vi "DynamicMotionMagicVoltage SetControl.vi"(0 "UseTimesync":bool, 1 "StopSendingOtherRequests":bool=TRUE, 2 "Position":dbl, 3 "Velocity":dbl, 4 "Acceleration":dbl, 5 "Jerk":dbl, 6 "EnableFOC":bool=TRUE, 7 "error in":errorcluster, 8 "FeedForward":dbl, 9 "Slot":i32, 10 "OverrideBrakeDurNeutral":bool, 11 "LimitForwardMotion":bool, 12 "LimitReverseMotion":bool, 13 "IgnoreHardwareLimits":bool, 18 "Update Frequency (Hz)":dbl=100.0) -> (20 "DeviceReference Out":T1, 27 "error out":errorcluster)   [LabVIEW 2023]
doc: "Requests Motion Magic® to target a final position using a motion profile. This dynamic request allows runtime changes to Cruise Velocity, Acceleration, and Jerk. Users can optionally provide a voltage feedforward. This control requires use of a CANivore.\nMotion Magic® produces a motion profile in real-time while attempting to honor the specified Cruise Velocity, Acceleration, and (optional) Jerk. This control mode does not use the Expo_kV or Expo_kA configs.\nTarget position can be changed on-the-fly and Motion Magic® will do its best to adjust the profile. This control mode is voltage-based, so relevant closed-loop gains will use Volts for the numerator."
uses:
  Users/test.DESKTOP-CORY/Documents/PhoenixProLabVIEWGeneration/CopyDown/DeviceReference.ctl
panel:
  in  "DeviceReference":T1
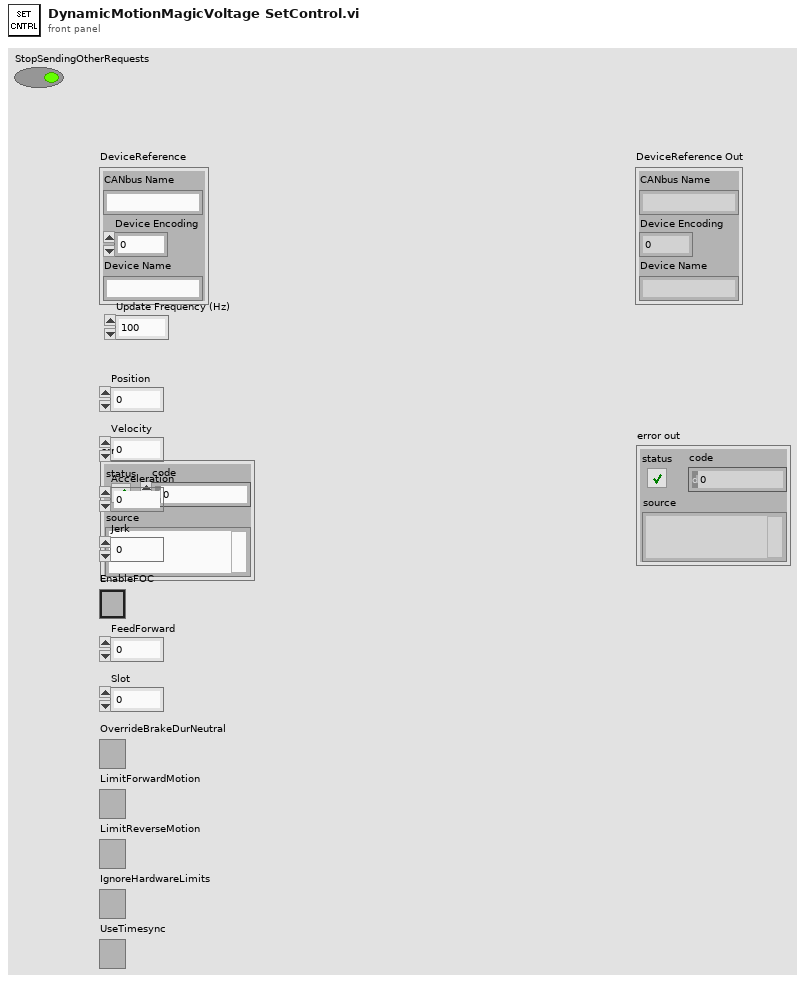
[diagram p1: front panel]
types:
  T1 = typedef "DeviceReference.ctl" = cluster{"CANbus Name":string, "Device Encoding":u32, "Device Name":string}
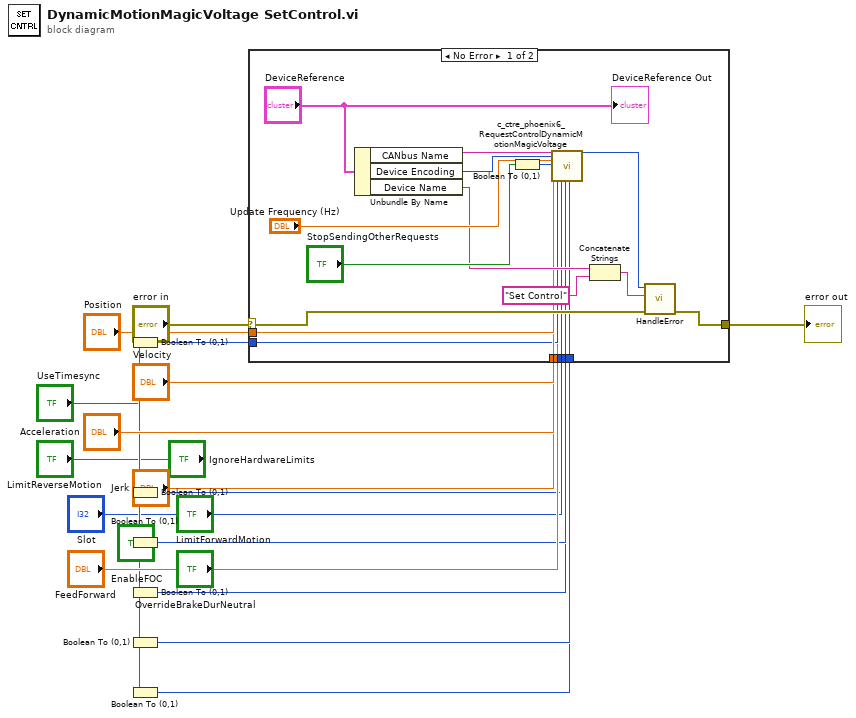
[diagram p0: block diagram]
diagram:
  n1 = Boolean To (0,1)(Boolean="EnableFOC") -> (0, 1=w13:i16)
  n2 = Boolean To (0,1)(Boolean="OverrideBrakeDurNeutral") -> (0, 1=w9:i16)
  n3 = Boolean To (0,1)(Boolean="LimitForwardMotion") -> (0, 1=w7:i16)
  n4 = Boolean To (0,1)(Boolean="LimitReverseMotion") -> (0, 1=w5:i16)
  n5 = Boolean To (0,1)(Boolean="IgnoreHardwareLimits") -> (0, 1=w3:i16)
  n6 = Boolean To (0,1)(Boolean="UseTimesync") -> (0, 1=w1:i16)
  n7 = case shown="No Error" "error in" {
    selector: "error in" -> [w37 w45]
    tunnel: [w36 w45] -> w19
    tunnel: "Position" -> [w32 _]
    tunnel: "Velocity" -> [w31 _]
    tunnel: "Acceleration" -> [w30 _]
    tunnel: "Jerk" -> [w29 _]
    tunnel: w13 -> [w28 _]
    tunnel: "FeedForward" -> [w27 _]
    tunnel: "Slot" -> [w26 _]
    tunnel: w9 -> [w25 _]
    tunnel: w7 -> [w24 _]
    tunnel: w5 -> [w23 _]
    tunnel: w3 -> [w22 _]
    tunnel: w1 -> [w21 _]
    frame No Error {
      n8 = Unbundle By Name("DeviceReference") -> ("CANbus Name"=w43:string, "Device Encoding"=w42:u32, "Device Name"=w35:string)
      n9 = Boolean To (0,1)(Boolean="StopSendingOtherRequests") -> (0, 1=w39:i16)
      n10 = call <vilib>:"c_ctre_phoenix6_RequestControlDynamicMotionMagicVoltage.vi"("String 2"=w43, "Numeric 2"=w42, "Numeric 3"="Update Frequency (Hz)", "Numeric 4"=w39, "Numeric 5"=w32, "Numeric 6"=w31, "Numeric 7"=w30, "Numeric 8"=w29, "Numeric 9"=w28, "Numeric 10"=w27, "Numeric 11"=w26, "Numeric 12"=w25, "Numeric 13"=w24, "Numeric 14"=w23, "Numeric 15"=w22, 15:w21) -> ("Numeric"=w38:i32)  [unwired: 10 in, 1 out]
      n11 = Concatenate Strings(w35, "Set Control" ("origin")) -> (w33:string)
      n12 = call "HandleError.vi"("error in"=w37, "origin"=w33, "Status"=w38) -> ("error out"=w36:errorcluster)  [unwired: 8 in]
      "DeviceReference Out" <- "DeviceReference"
    }
    frame Error {
    }
  }
  "error out" <- w19
